vi "FCI Bin Test_Lip.vi"(8 "error in (no error)":errorcluster, 11 "Image 3":T1) -> (0 "error IO":errorcluster, 1 "Lip outer width":sgl format="%.2f", 2 "Box Width":sgl)   [LabVIEW 2019, in "Algorithm.lvclass"]
uses:
  FrameworkOverrides/Algorithm.lvclass
  <vilib>/vision/NI_Vision_Development_Module.lvlib
  <vilib>/vision/Measure.llb/Straight Edge Process.ctl
  <vilib>/vision/Measure.llb/Straight Edge Options.ctl
  <vilib>/vision/Measure.llb/Edge Polarity.ctl
  <vilib>/vision/Measure.llb/Edge Options.ctl
  <vilib>/vision/Image Controls.llb/IMAQ Image.ctl
panel:
  out "Angle (Pixel)":dbl
  in  "Y coord lower limit":dbl=350.0 format="%#_13g"
  in  "Y coord upper limit":dbl=730.0 format="%#_13g"
  out "Y Coord":dbl[](array[numeric])
  out "Number of Particles":i32
  out "subarray 2":dbl[](array[numeric])
  out "index of element":i32
  out "Array":bool[](array[boolean])
  out "X Coord":dbl[](array[numeric])
  out "Image 2":T1(plugin-control)
  out "Image":T1(plugin-control)
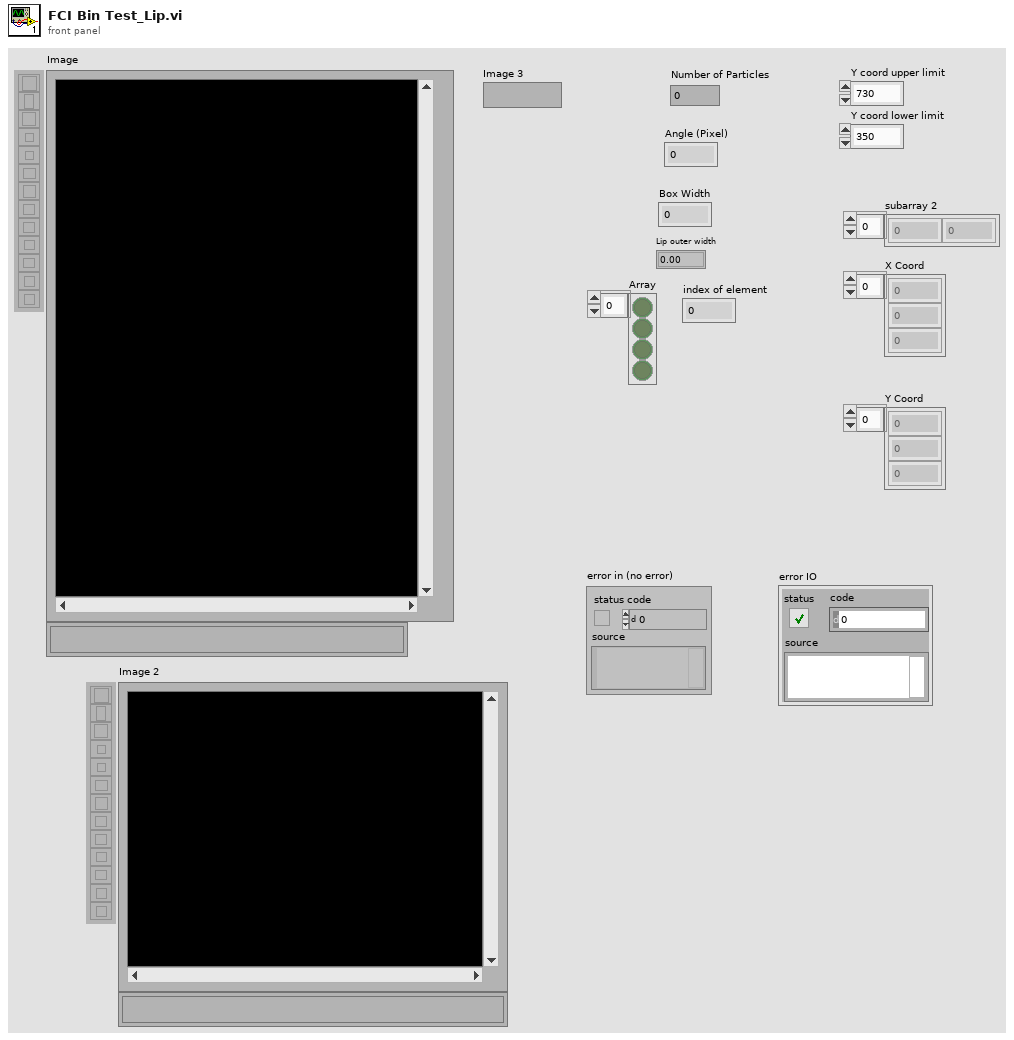
[diagram p1: front panel]
types:
  T1 = typedef "IMAQ Image.ctl" = refnum<image>
  T2 = typedef "Edge Options.ctl" = cluster{"Edge Polarity":T3, "Kernel Size":u32, "Width":u32, "Minimum Edge Strength":sgl, "Interpolation Type":enum32{"Zero Order", "Bilinear", "Quadratic", "Cubic", "Bilinear Fixed"}, "Data Processing Method":enum32{"Average", "Median"}}
  T3 = typedef "Edge Polarity.ctl" = u32
  T4 = cluster{"Left":dbl, "Top":dbl, "Right":dbl, "Bottom":dbl, "Angle":dbl}
  T5 = cluster{"Search Direction":u32, "Edge Options":T2, "Show Search Area":bool, "Show Search Lines":bool, "Show Edges Found":bool, "Show Result":bool, "Search Area Color":u32, "Search Lines Color":u32, "Edge Locations Color":u32, "Result Color":u32, "Overlay Group Name":string}
  T6 = typedef "Straight Edge Options.ctl" = cluster{"Number of Lines":i32, "Type":T7, "Min. Score":dbl, "Max. Score":dbl, "Orientation":dbl, "Angle Range":dbl, "Angle Tolerance":dbl, "Step Size":u32, "Min. SNR (db)":dbl, "Min. Points (%)":dbl, "Hough Iterations":i32}
  T7 = typedef "Straight Edge Process.ctl" = enum32{"First Edge Rake", "Best Edge Rake", "Hough Edge Rake", "First Edge Projection", "Best Edge Projection"}
  T8 = enum16{"Get First Edge", "Get First + Last Edge", "Get All Edges", "Get Best Edge"}
  T9 = typedef "Particle Parameters" = i32
  T10 = cluster{"Measurement Parameter":T9, "Range Lower Value":dbl, "Range Upper Value":dbl, "Range":bool, "Measurement Type":bool}[]
  T11 = typedef "Image Type" = u32
  T12 = typedef "ROI Descriptor" = cluster{"Global Rectangle":i32[], "Contours":cluster{"ID":enum32{"External", "Internal"}, "Type":u32, "Coordinates":i32[]}[]}
  T13 = cluster{"Point1 (Pixels)":cluster{"X":sgl, "Y":sgl}, "Point2 (Pixels)":cluster{"X":sgl, "Y":sgl}, "Point1 (Real-World)":cluster{"X":sgl, "Y":sgl}, "Point2 (Real-World)":cluster{"X":sgl, "Y":sgl}, "Angle (Pixel)":dbl, "Angle (Real-World)":dbl, "Score":dbl, "Straightness":dbl, "Average SNR (db)":dbl, "Calibration Valid":bool}[]
  T14 = cluster{"Point1 (Pixels)":cluster{"X":sgl, "Y":sgl}, "Point2 (Pixels)":cluster{"X":sgl, "Y":sgl}, "Point1 (Real-World)":cluster{"X":sgl, "Y":sgl}, "Point2 (Real-World)":cluster{"X":sgl, "Y":sgl}, "Angle (Pixel)":dbl, "Angle (Real-World)":dbl, "Score":dbl, "Straightness":dbl, "Average SNR (db)":dbl, "Calibration Valid":bool}
  T15 = typedef "Edge New.ctl" = cluster{"Location (Pixel)":cluster{"X":sgl, "Y":sgl}, "Location (Real-World)":cluster{"X":sgl, "Y":sgl}, "Distance (Pixel)":dbl, "Distance (Real-World)":dbl, "Strength":dbl, "Noise":dbl, "Rising?":bool}
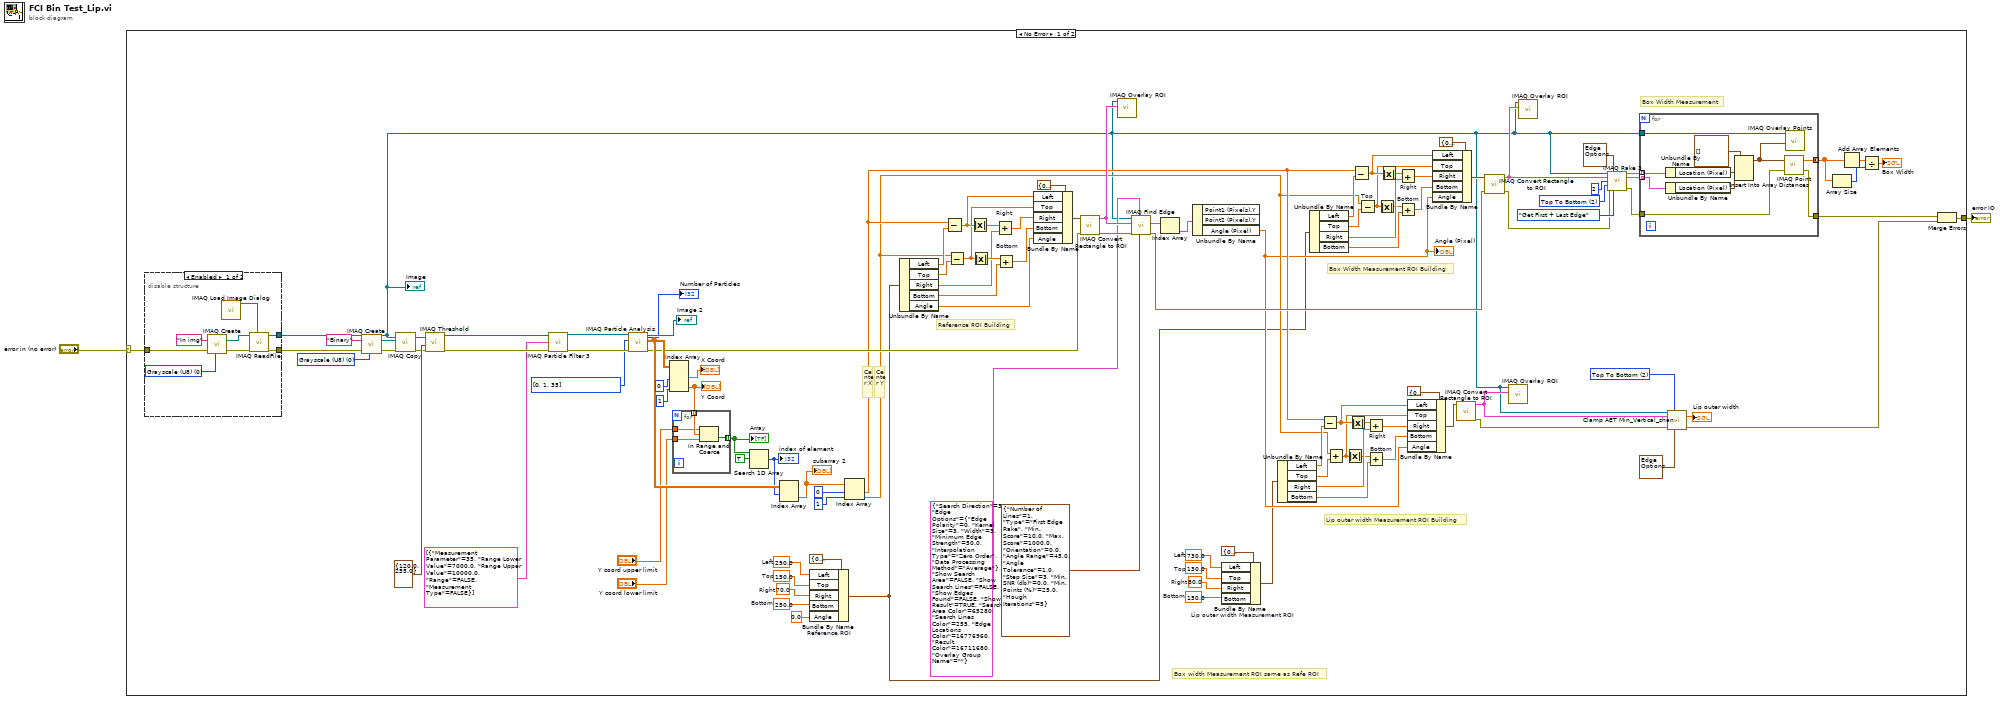
[diagram p0: block diagram]
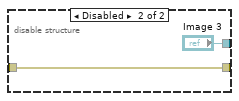
[diagram p2: hidden frame]
diagram:
  n1 = case shown="No Error" "error in (no error)" {
    selector: "error in (no error)" -> [w38 w140]
    tunnel: [w17 w140] -> w1
    frame No Error {
      w5 = u16 2 items=["Left To Right", "Right To Left", "Top To Bottom", "Bottom To Top"] ("Scanning axis")
      w13 = 150.0  # Bottom
      w14 = 80.0  # Right
      w15 = 130.0  # Top
      w16 = 730.0  # Left
      w46 = 250.0  # Bottom
      w47 = 70.0  # Right
      w48 = 150.0  # Top
      w49 = 290.0  # Left
      w80 = u16 2 items=["Left To Right", "Right To Left", "Top To Bottom", "Bottom To Top"] ("Scan Direction")
      w107 = T9[] [0, 1, 35] items=["Center of Mass X", "Center of Mass Y", "First Pixel X", "First Pixel Y", "Bounding Rect Left", "Bounding Rect Top", "Bounding Rect Right", "Bounding Rect Bottom", "Max Feret Diameter Start X", "Max Feret Diameter Start Y", "Max Feret Diameter End X", "Max Feret Diameter End Y", "Max Horiz. Segment Length Left", "Max Horiz. Segment Length Right", "Max Horiz. Segment Length Row", "-", "Bounding Rect Width", "Bounding Rect Height", "Bounding Rect Diagonal", "Perimeter", "Convex Hull Perimeter", "Holes' Perimeter", "Max Feret Diameter", "Equivalent Ellipse Major Axis", "Equivalent Ellipse Minor Axis", "Equivalent Ellipse Minor Axis (Feret)", "Equivalent Rect Long Side", "Equivalent Rect Short Side", "Equivalent Rect Diagonal", "Equivalent Rect Short Side (Feret)", "Average Horiz. Segment Length", "Average Vert. Segment Length", "Hydraulic Radius", "Waddel Disk Diameter", "-", "Area", "Holes' Area", "Particle & Holes' Area", "Convex Hull Area", "Image Area", "-", "Number of Holes", "Number of Horiz. Segments", "Number of Vert. Segments", "-", "Orientation", "Max Feret Diameter Orientation", "-", "% Area/Image Area", "% Area/(Particle & Holes' Area)", "Ratio of Equivalent Ellipse Axes", "Ratio of Equivalent Rect Sides", "-", "Elongation Factor", "Compactness Factor", "Heywood Circularity Factor", "Type Factor", "-", "Sum X", "Sum Y", "Sum XX", "Sum XY", "Sum YY", "Sum XXX", "Sum XXY", "Sum XYY", "Sum YYY", "-", "Moment of Inertia XX", "Moment of Inertia XY", "Moment of Inertia YY", "Moment of Inertia XXX", "Moment of Inertia XXY", "Moment of Inertia XYY", "Moment of Inertia YYY", "Norm. Moment of Inertia XX", "Norm. Moment of Inertia XY", "Norm. Moment of Inertia YY", "Norm. Moment of Inertia XXX", "Norm. Moment of Inertia XXY", "Norm. Moment of Inertia XYY", "Norm. Moment of Inertia YYY", "Hu Moment 1", "Hu Moment 2", "Hu Moment 3", "Hu Moment 4", "Hu Moment 5", "Hu Moment 6", "Hu Moment 7"] ("Pixel Measurements")
      w114 = T11 0 items=["Grayscale (U8)", "Grayscale (I16)", "Grayscale (SGL)", "Complex (CSG)", "RGB (U32)", "HSL (U32)", "RGB (U64)", "Grayscale (U16)"] ("Image Type")
      # "Lip outer width Measurement ROI Building"
      # "Box width Measurement ROI same as Refe ROI"
      # "Box Width Measurement"
      # "Box Width Measurement ROI Building"
      # "Reference ROI Building"
      # "Center Y"
      # "Center X"
      n2 = disable-structure shown="Enabled" {
        disable-tunnel: [w119 w125] -> w67
        disable-tunnel: w38 -> [w117 w125]
        disable-tunnel: [w116 "Image 3"] -> w6
        frame Enabled {
          w121 = T11 0 items=["Grayscale (U8)", "Grayscale (I16)", "Grayscale (SGL)", "Complex (CSG)", "RGB (U32)", "HSL (U32)", "RGB (U64)", "Grayscale (U16)"] ("Image Type")
          n3 = call "IMAQ Create"("Image Name"="In img", "Image Type"=w121, "error in (no error)"=w117) -> ("New Image"=w123:T1, "error out"=w120:errorcluster)  [unwired: 2 in]
          n4 = call "IMAQ Load Image Dialog"() -> ("Path"=w118:path)  [unwired: 9 in, 2 out]
          n5 = call "IMAQ ReadFile"("File Path"=w118, "error in (no error)"=w120, "Image"=w123) -> ("error out"=w119:errorcluster, "Image Out"=w116:T1)  [unwired: 4 in, 3 out]
        }
        frame Disabled {
        }
      }
      "Image" <- w6
      n6 = call "IMAQ Create"("Image Name"="Binary", "Image Type"=w114, "error in (no error)"=w67) -> ("New Image"=w113:T1, "error out"=w112:errorcluster)  [unwired: 2 in]
      n7 = call "IMAQ Copy"("error in (no error)"=w112, "Image Dst"=w113, "Image Src"=w6) -> ("error out"=w40:errorcluster, "Image Dst Out"=w69:T1)  [unwired: 3 in]
      n8 = call "IMAQ Threshold"("error in (no error)"=w40, "Range"=cluster{"Lower value":sgl, "Upper value":sgl} {"Lower value"=120.0, "Upper value"=255.0}, "Image Src"=w69) -> ("error out"=w111:errorcluster, "Image Dst Out"=w110:T1)  [unwired: 7 in]
      n9 = call "IMAQ Particle Filter 3"("Image Src"=w110, "Selection Values"=T10 [{"Measurement Parameter"=35, "Range Lower Value"=7000.0, "Range Upper Value"=10000.0, "Range"=FALSE, "Measurement Type"=FALSE}], "error in (no error)"=w111) -> ("Image Dst Out"=w109:T1, "error out"=w108:errorcluster)  [unwired: 10 in, 1 out]
      n10 = call "IMAQ Particle Analysis"("error in (no error)"=w108, "Pixel Measurements"=w107, "Image"=w109) -> ("error out"=w39:errorcluster, "Particle Measurements (Pixels)"=w63:dbl[][], "Image Out (duplicate)"=→"Image 2":T1, "Number of Particles"=→"Number of Particles":i32)  [unwired: 3 in, 2 out]
      n11 = Index Array(array=w63, index (col) #1=0 ("disabled index (col)"), index (col) #2=1 ("index (col)")) -> (element #1=→"X Coord":dbl[], element #2=w55:dbl[])  [unwired: 2 in]
      "Y Coord" <- w55
      n12 = for {
        tunnel: w55 -> [w129] mode=indexing
        tunnel: [w128] -> w65 mode=indexing
        tunnel: "Y coord upper limit" -> [w127]
        tunnel: "Y coord lower limit" -> [w126]
        n13 = In Range and Coerce(upper limit=w127, x=w129, lower limit=w126) -> (In Range?=w128:bool)  [unwired: 1 out]
      }
      "Array" <- w65
      n14 = Search 1D Array(1D array=w65, element=TRUE) -> (index of element=w62:i32)  [unwired: 1 in]
      "index of element" <- w62
      n15 = Index Array(array=w63, index (row)=w62) -> (element=w61:dbl[])  [unwired: 1 in]
      "subarray 2" <- w61
      n16 = Bundle By Name "Reference ROI"(cluster=T4 {"Left"=0.0, "Top"=0.0, "Right"=0.0, "Bottom"=0.0, "Angle"=0.0} ("input cluster"), "Left"=w49, "Top"=w48, "Right"=w47, "Bottom"=w46, "Angle"=0.0) -> (w10:T4)
      n17 = Index Array(array=w61, index #1=0 ("index"), index #2=1 ("index")) -> (element #1=w21:dbl, element #2=w20:dbl)
      n18 = Unbundle By Name(w10) -> ("Left"=w90:dbl, "Top"=w89:dbl, "Right"=w88:dbl, "Bottom"=w87:dbl, "Angle"=w86:dbl)
      n19 = Subtract(x=w21, y=w90) -> (x-y=w98:dbl)
      n20 = Subtract(x=w20, y=w89) -> (x-y=w97:dbl)
      n21 = Absolute Value(x=w98) -> (abs(x)=w101:dbl)
      n22 = Absolute Value(x=w97) -> (abs(x)=w100:dbl)
      n23 = Add "Right"(x=w101, y=w88) -> (x+y=w96:dbl)
      n24 = Add "Bottom"(x=w100, y=w87) -> (x+y=w95:dbl)
      n25 = Bundle By Name(cluster=T4 {"Left"=0.0, "Top"=0.0, "Right"=0.0, "Bottom"=0.0, "Angle"=0.0} ("input cluster"), "Left"=w98, "Top"=w97, "Right"=w96, "Bottom"=w95, "Angle"=w86) -> (w72:T4)
      n26 = call "IMAQ Convert Rectangle to ROI"("error in (no error)"=w39, "Rectangle"=w72) -> ("error out"=w85:errorcluster, "ROI Descriptor"=w43:T12)  [unwired: 7 in]
      n27 = call "IMAQ Overlay ROI"("ROI Descriptor"=w43, "Image"=w6) -> ()  [unwired: 8 in, 2 out]
      n28 = call "IMAQ Find Edge"("Line Fit Options"=T6 {"Number of Lines"=1, "Type"=enum."First Edge Rake", "Min. Score"=10.0, "Max. Score"=1000.0, "Orientation"=0.0, "Angle Range"=45.0, "Angle Tolerance"=1.0, "Step Size"=3, "Min. SNR (db)"=0.0, "Min. Points (%)"=25.0, "Hough Iterations"=5}, "Options"=T5 {"Search Direction"=3, "Edge Options"={"Edge Polarity"=0, "Kernel Size"=3, "Width"=3, "Minimum Edge Strength"=50.0, "Interpolation Type"=enum."Zero Order", "Data Processing Method"=enum."Average"}, "Show Search Area"=FALSE, "Show Search Lines"=FALSE, "Show Edges Found"=FALSE, "Show Result"=TRUE, "Search Area Color"=65280, "Search Lines Color"=255, "Edge Locations Color"=16776960, "Result Color"=16711680, "Overlay Group Name"=""}, "error in (no error)"=w85, "ROI Descriptor"=w43, "Image"=w6) -> ("error out"=w37:errorcluster, "Straight Edges"=w83:T13)  [unwired: 3 in, 2 out]
      n29 = Index Array(array=w83) -> (element=w82:T14)  [unwired: 1 in]
      n30 = Unbundle By Name(w82) -> ("Angle (Pixel)"=w19:dbl)  [unwired: 2 out]
      "Angle (Pixel)" <- w19
      n31 = Bundle By Name "Lip outer width Measurement ROI"(cluster=T4 {"Left"=0.0, "Top"=0.0, "Right"=0.0, "Bottom"=0.0, "Angle"=0.0} ("input cluster"), "Left"=w16, "Top"=w15, "Right"=w14, "Bottom"=w13) -> (w11:T4)
      n32 = Unbundle By Name(w11) -> ("Left"=w28:dbl, "Top"=w27:dbl, "Right"=w26:dbl, "Bottom"=w25:dbl)
      n33 = Unbundle By Name(w10) -> ("Left"=w94:dbl, "Top"=w93:dbl, "Right"=w92:dbl, "Bottom"=w91:dbl)
      n34 = Subtract(x=w21, y=w28) -> (x-y=w31:dbl)
      n35 = Add(x=w20, y=w27) -> (x+y=w23:dbl)
      n36 = Absolute Value(x=w23) -> (abs(x)=w24:dbl)
      n37 = Absolute Value(x=w31) -> (abs(x)=w33:dbl)
      n38 = Subtract(x=w21, y=w94) -> (x-y=w104:dbl)
      n39 = Subtract "Top"(x=w20, y=w93) -> (x-y=w51:dbl)
      n40 = Add "Right"(x=w33, y=w26) -> (x+y=w30:dbl)
      n41 = Add "Bottom"(x=w24, y=w25) -> (x+y=w29:dbl)
      n42 = Absolute Value(x=w51) -> (abs(x)=w52:dbl)
      n43 = Absolute Value(x=w104) -> (abs(x)=w106:dbl)
      n44 = Add "Right"(x=w106, y=w92) -> (x+y=w103:dbl)
      n45 = Add "Bottom"(x=w52, y=w91) -> (x+y=w102:dbl)
      n46 = Bundle By Name(cluster=T4 {"Left"=0.0, "Top"=0.0, "Right"=0.0, "Bottom"=0.0, "Angle"=0.0} ("input cluster"), "Left"=w31, "Top"=w23, "Right"=w30, "Bottom"=w29, "Angle"=w19) -> (w22:T4)
      n47 = Bundle By Name(cluster=T4 {"Left"=0.0, "Top"=0.0, "Right"=0.0, "Bottom"=0.0, "Angle"=0.0} ("input cluster"), "Left"=w104, "Top"=w51, "Right"=w103, "Bottom"=w102, "Angle"=w19) -> (w71:T4)
      n48 = call "IMAQ Convert Rectangle to ROI"("Rectangle"=w22) -> ("error out"=w9:errorcluster, "ROI Descriptor"=w7:T12)  [unwired: 8 in]
      n49 = call "IMAQ Convert Rectangle to ROI"("error in (no error)"=w37, "Rectangle"=w71) -> ("error out"=w36:errorcluster, "ROI Descriptor"=w50:T12)  [unwired: 7 in]
      n50 = call "IMAQ Overlay ROI"("ROI Descriptor"=w7, "Image"=w6) -> ()  [unwired: 8 in, 2 out]
      n51 = call "IMAQ Overlay ROI"("ROI Descriptor"=w50, "Image"=w6) -> ()  [unwired: 8 in, 2 out]
      n52 = call "IMAQ Rake 3"("Image"=w6, "Edge Options"=T2 {"Edge Polarity"=0, "Kernel Size"=5, "Width"=5, "Minimum Edge Strength"=50.0, "Interpolation Type"=enum."Zero Order", "Data Processing Method"=enum."Average"}, "ROI Descriptor"=w50, "Step Size"=u32 2, "Scan Direction"=w80, "error in (no error)"=w36, "Process"=T8."Get First + Last Edge") -> ("First Edges"=w77:T15[], "Last Edges"=w68:T15[], "error out"=w35:errorcluster)  [unwired: 5 in, 1 out]
      n53 = for {
        tunnel: w77 -> [w139] mode=indexing
        tunnel: w68 -> [w138] mode=indexing
        tunnel: [w136] -> w76 mode=concatenating
        tunnel: w6 -> [w132]
        tunnel: w35 -> [w131]
        tunnel: [w130] -> w18
        n54 = Unbundle By Name(w139) -> ("Location (Pixel)"=w134:cluster{"X":sgl, "Y":sgl})
        n55 = Unbundle By Name(w138) -> ("Location (Pixel)"=w135:cluster{"X":sgl, "Y":sgl})
        n56 = Insert Into Array(array=cluster{"X":sgl, "Y":sgl}[] [], new element #1=w134, new element #2=w135) -> (w133:cluster{"X":sgl, "Y":sgl}[])  [unwired: 1 in]
        n57 = call "IMAQ Point Distances"("Points"=w133, "error in (no error)"=w131) -> ("Distances"=w136:sgl[], "error out"=w130:errorcluster)  [unwired: 3 in]
        n58 = call "IMAQ Overlay Points"("Array of Points"=w133, "Image"=w132) -> ()  [unwired: 8 in, 2 out]
      }
      n59 = call "Clamp AET Min_Vertical_shan.vi"("Image"=w6, "Scanning axis"=w5, "ROI Descriptor"=w7, "error in (no error)"=w9, "Edge Options"=T2 {"Edge Polarity"=0, "Kernel Size"=3, "Width"=3, "Minimum Edge Strength"=50.0, "Interpolation Type"=enum."Bilinear Fixed", "Data Processing Method"=enum."Average"}) -> ("Distance"=→"Lip outer width":sgl, "error out"=w8:errorcluster)  [unwired: 4 in, 5 out]
      n60 = Array Size(array=w76) -> (size(s)=w74:i32)
      n61 = Add Array Elements(numeric array=w76) -> (sum=w75:sgl)
      n62 = Divide(x=w75, y=w74) -> (x/y=→"Box Width":sgl)
      n63 = Merge Errors(w18, w8) -> (w17:errorcluster)
    }
    frame Error {
    }
  }
  "error IO" <- w1
